vi "flattenAccelerationToXML_Scalar.vi"(8 "error in (no error)":errorcluster, 9 "accelerationUnitInXML":T1, 10 "accelerationAgain":variant, 11 "acceleration":dbl[unit]) -> (0 "error out":errorcluster, 3 "xmlString":string)   [LabVIEW 2016, in "UnitsAndXML.lvlib"]
uses:
  <userlib>/Common/UnitsAndXML/UnitsAndXML.lvlib
  <userlib>/Common/UnitsAndXML/FlattenItemWithUnitToXML/FlattenAccelerationToXML/AccelerationUnit.ctl
  <vilib>/Utility/VariantDataType/VariantType.lvlib
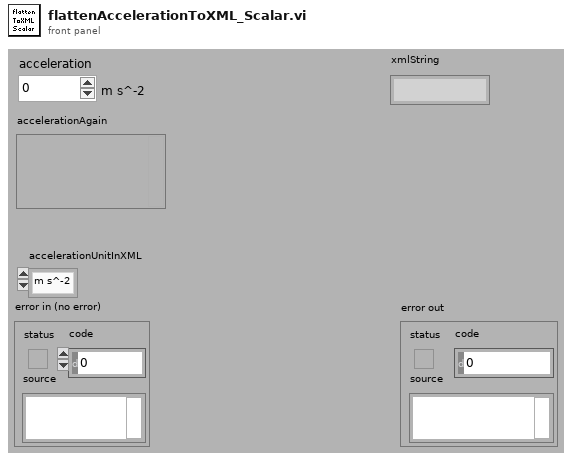
[diagram p1: front panel]
types:
  T1 = typedef "UnitsAndXML.lvlib/AccelerationUnit.ctl" = enum16{"m s^-2"}
  T2 = typedef "VariantType.lvlib/Type.ctl" = enum8{"Invalid Type", "Void", "I8", "I16", "I32", "I64", "U8", "U16", "U32", "U64", "Single Float", "Double Float", "Extended Float", "Single Complex", "Double Complex", "Extended Complex", "Enum U8", "Enum U16", "Enum U32", "Enum U64", "Single Float With Unit", "Double Float With Unit", "Extended Float With Unit", "Single Complex with Unit", "Double Complex with Unit", "Extended Complex with Unit", "Boolean", "String", "Path", "Picture", "Tag", "Array", "Cluster", "Variant", "LV Variant", "Waveform", "Timestamp", "Digital Waveform", "Digital Data", "ExpressData", "Refnum", "External Data", "VI", "Poly VI", "LabVIEW Class Instance", "Fixed Point"}
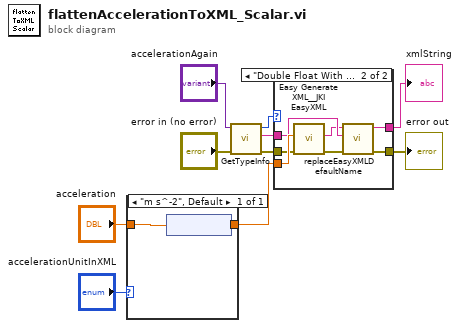
[diagram p0: block diagram]
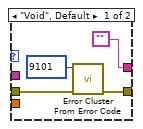
[diagram p2: hidden frame]
diagram:
  n1 = case shown="\"m s^-2\", Default" "accelerationUnitInXML" {
    tunnel: "acceleration" -> [w12]
    tunnel: [w11] -> w10
    frame "m s^-2", Default {
      n2 = node(w12) -> (w11:dbl)
    }
  }
  n3 = call <vilib>:"GetTypeInfo.vi"("error in (no error)"="error in (no error)", "Variant"="accelerationAgain") -> ("error out"=w2:errorcluster, "Name"=w1:string, "Type Enum"=w3:T2)  [unwired: 5 in, 2 out]
  n4 = case shown="\"Double Float With Unit\"" w3 {
    tunnel: w10 -> [_ w23]
    tunnel: ["" w22] -> w7
    tunnel: [w15 w21] -> w6
    tunnel: w2 -> [w13 w18]
    tunnel: w1 -> [_ w20]
    frame "Void", Default {
      n5 = call <vilib>:"Error Cluster From Error Code.vi"("error in (no error)"=w13, "error code (0)"=9101) -> ("error out"=w15:errorcluster)  [unwired: 7 in]
    }
    frame "Double Float With Unit" {
      n6 = call <vilib>:"Easy Generate XML__JKI EasyXML.vi"("error in (no error)"=w18, "LabVIEW Data"=w23) -> ("error out"=w17:errorcluster, "XML String"=w19:string)  [unwired: 8 in]
      n7 = call <userlib>:"replaceEasyXMLDefaultName.vi"("error in"=w17, "desiredName"=w20, "easyXMLStringWithDefaultNames"=w19) -> ("error out"=w21:errorcluster, "xmlString"=w22:string)  [unwired: 7 in]
    }
  }
  "xmlString" <- w7
  "error out" <- w6
